vi "Anlagenuebersicht_amium2.vi"() -> ()   [LabVIEW 2020, in "Amium PNS.lvlib"]
uses:
  Amium PNS.lvlib
  PNS Istwerte_Amium.ctl
  Visualisierungs Elemente/String - Ausgabefeld.ctl
  Amium Zustand.ctl
  Seiten/System Einstellungen V2/Aktioen FGV System.ctl
  Aktion FGV Amium Daten.ctl
  Allgemein/allgemeine Sub-VIs.lvlib
  Seiten/System Einstellungen V2/System Einstellungen V2.lvlib
panel:
  in  "Amium Zustände 2":T1 items=["Pause", "Aufheizphase", "Standby", "Messen", "Spülen", "Leakcheck"]
  out "Amium Zustände":T2
  in  "4 - Fach":bool
  in  "10-Fach":bool
  out "IN10":bool caption="TG"
  out "IN10 2":bool caption="Ex"
  out "IN9":bool caption="TG"
  out "IN9 2":bool caption="Ex"
  out "IN8":bool caption="TG"
  out "IN8 2":bool caption="Ex"
  out "IN7":bool caption="TG"
  out "IN7 2":bool caption="Ex"
  out "IN6":bool caption="TG"
  out "IN6 2":bool caption="Ex"
  out "IN3":bool caption="TG"
  out "IN3 2":bool caption="Ex"
  out "IN4":bool caption="TG"
  out "IN4 2":bool caption="Ex"
  out "AA":bool caption="TG"
  out "Purge":bool caption="Ex"
  out "IN5":bool caption="TG"
  out "IN5 2":bool caption="Ex"
  out "IN1":bool caption="TG"
  out "IN1 2":bool caption="Ex"
  out "IN2":bool caption="TG"
  out "IN2 2":bool caption="Ex"
  out "EX":bool caption="TG"
  out "EX2":bool caption="Ex"
  out "PNS Istwerte":T3 {"Istwert 14" format="%.1f"; "Istwert 13" format="%.1f"; "Istwert 12" format="%.1f"; "Istwert 11" format="%.1f"; "Istwert 10" format="%.1f"; "Istwert 9" format="%.1f"; "Istwert 8" format="%.1f"; "Istwert 7" format="%.1f"; "Istwert 6" format="%.1f"; "Istwert 5" format="%.1f"; "Istwert 4" format="%.1f"; "Istwert 3" format="%.1f"; "Istwert 2" format="%.1f"; "Istwert 1" format="%.1f"}
  out "TG2":bool caption="Ex"
  out "TG":bool
  out "Bild":u16(ring)
  # "Pneumatikplan"
  # "Heizkreis 1:"
  # "Heizkreis 2:"
  # "Heizkreis 3:"
  # "Heizkreis 4:"
  # "Heizkreis 5:"
  # "Heizkreis 6:"
  # "Heizkreis 7:"
  # "Heizkreis 8:"
  # "Heizkreis 9:"
  # "Heizkreis 10:"
  # "Ofen / Filter:"
  # "HL Zuleitung:"
  # "Wanddurch-\nführung:"
  # "AddOn"
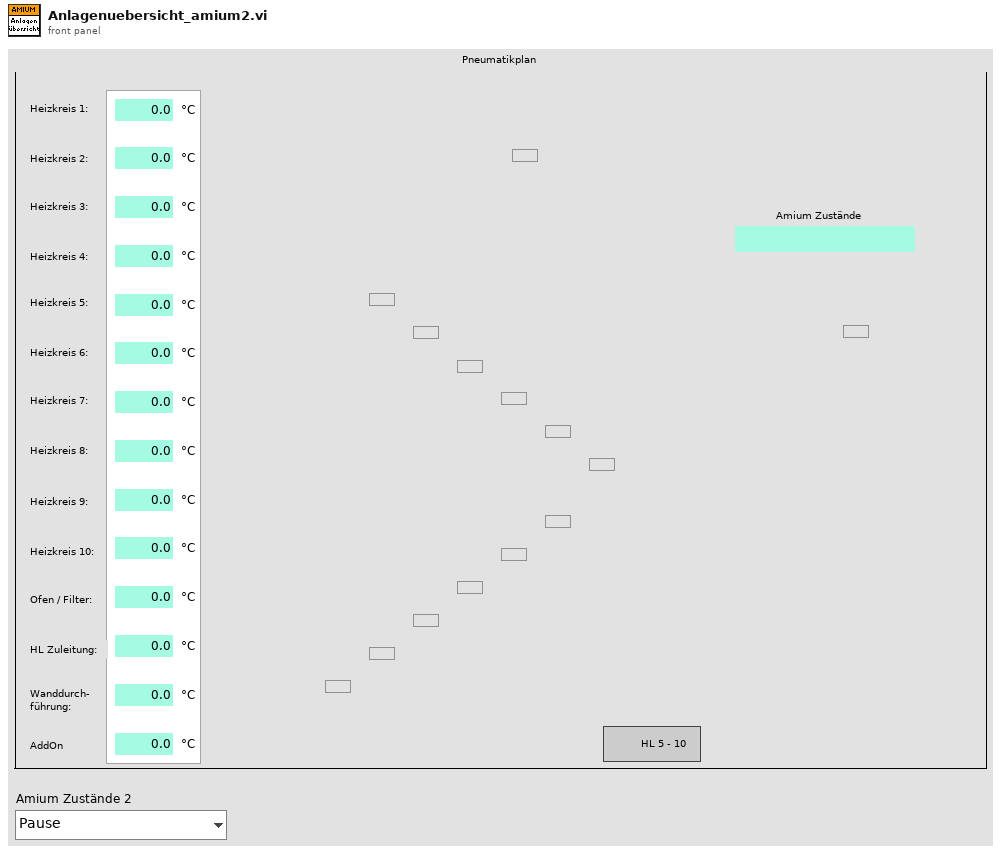
[diagram p1: front panel]
types:
  T1 = typedef "Amium PNS.lvlib/Amium Zustand.ctl" = u16
  T2 = typedef "String - Ausgabefeld.ctl" = string
  T3 = typedef "Amium PNS.lvlib/PNS Istwerte_Amium.ctl" = cluster{"Istwert 1":sgl, "Istwert 2":sgl, "Istwert 3":sgl, "Istwert 4":sgl, "Istwert 5":sgl, "Istwert 6":sgl, "Istwert 7":sgl, "Istwert 8":sgl, "Istwert 9":sgl, "Istwert 10":sgl, "Istwert 11":sgl, "Istwert 12":sgl, "Istwert 13":sgl, "Istwert 14":sgl}
  T4 = typedef "System Einstellungen V2.lvlib/Aktioen FGV System.ctl" = enum16{"lesen", "laden", "speichern", "Optionen schreiben", "Zeitstempel", "Reset BMP", "Reset SQP", "Wartung", "Werkseinstellung"}
  T5 = enum8{"Enabled", "Disabled", "Disabled and Grayed Out"}
  T6 = typedef "System Einstellungen V2.lvlib/Optionen.ctl" = cluster{"Störmeldep.":bool, "Betriebszustände":bool, "AK in ppm":bool, "log Cal-Gas":bool, "log 0-Gas":bool, "Durchflusssensor 0-5V":bool, "PNS?":bool, "Mit N2 spülen":bool, "TRE08":bool, "Amium 10-Fach":bool, "Verticale Scrollbar aktiv":bool, "Loggingtakt":bool, "AK Rezeptwechsel gleich wie MKS":bool, "NG ECO":bool}
  T7 = typedef "Amium PNS.lvlib/Aktion FGV Amium Daten.ctl" = enum16{"lesen", "Komm Daten", "Daten", "Error", "Regler", "Grenzwerte", "laden", "speichern"}
  T8 = typedef "Amium PNS.lvlib/Amium Anlagengrenzwerte PNS.ctl" = cluster{"Filter:":T9, "Ventilplatte:":T9, "Heizleitung 1:":T9, "Heizleitung 2:":T9, "Heizleitung 3:":T9, "Heizleitung 4:":T9, "Heizleitung 5:":T9, "Heizleitung 6:":T9, "Heizleitung 7:":T9, "Heizleitung 8:":T9, "Heizleitung 9:":T9, "Heizleitung 10:":T9, "Heizleitung 11:":T9, "Heizleitung 12:":T9}
  T9 = typedef "Amium PNS.lvlib/Amium Anlagengrenzwerte-Parameter Anzeige.ctl" = cluster{"Sollwert":T10, "Warn-Min":T10, "Warn-Max":T10, "Abschalt-Min":T10, "Abschalt-Max":T10, "Regler":u16}
  T10 = typedef "Zahlen-Eingabefeld.ctl" = sgl
  T11 = typedef "Amium PNS.lvlib/Daten Cluster.ctl" = cluster{"Amium Zustände":T1, "Samplepoint am PNS":i16, "Gerätekennung":string, "aktiver Samplepoint":i16[], "Messgasdruck":sgl}
  T12 = typedef "Amium PNS.lvlib/Temperaturregler Cluster.ctl" = cluster{"Istwert":sgl, "Sollwert":sgl, "Stellgröße":sgl, "Status":sgl, "Error":sgl}
  T13 = cluster{"Istwert":sgl, "Istwert":sgl, "Istwert":sgl, "Istwert":sgl, "Istwert":sgl, "Istwert":sgl, "Istwert":sgl, "Istwert":sgl, "Istwert":sgl, "Istwert":sgl, "Istwert":sgl, "Istwert":sgl, "Istwert":sgl, "Istwert":sgl}
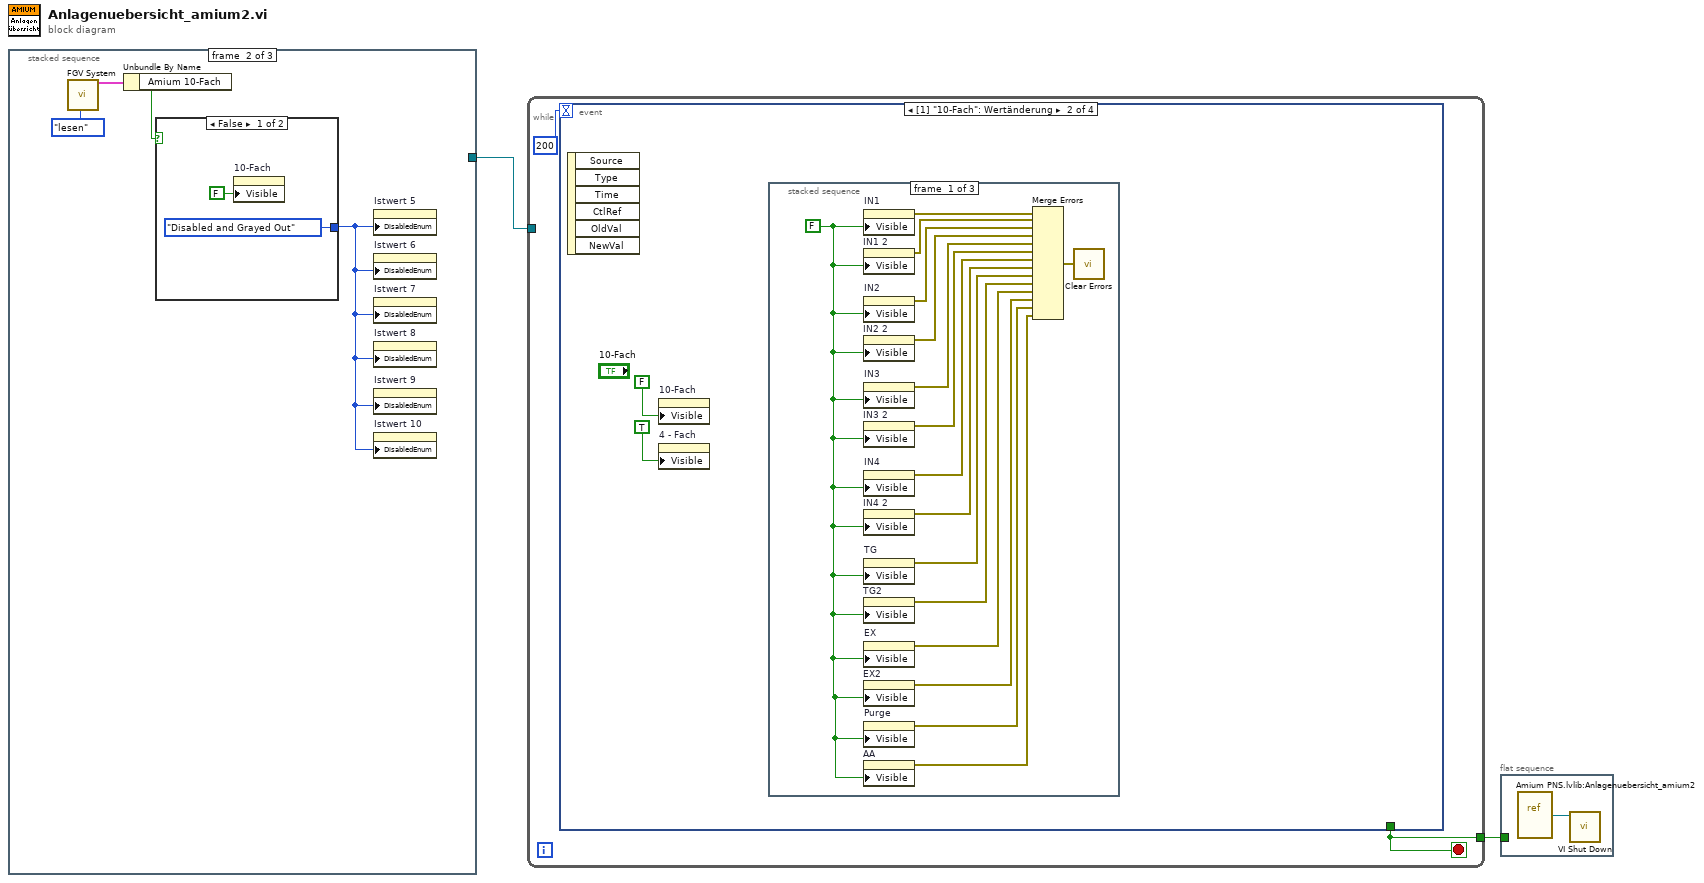
[diagram p0: block diagram]
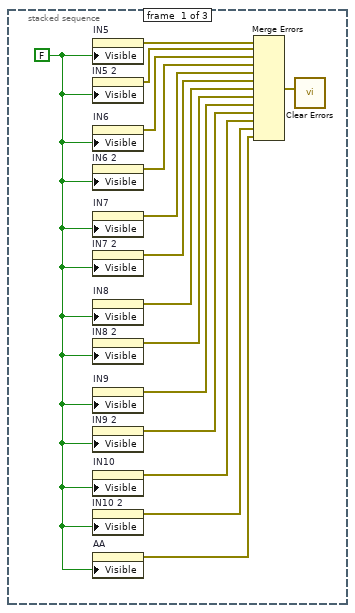
[diagram p2: hidden frame]
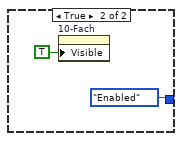
[diagram p3: hidden frame]
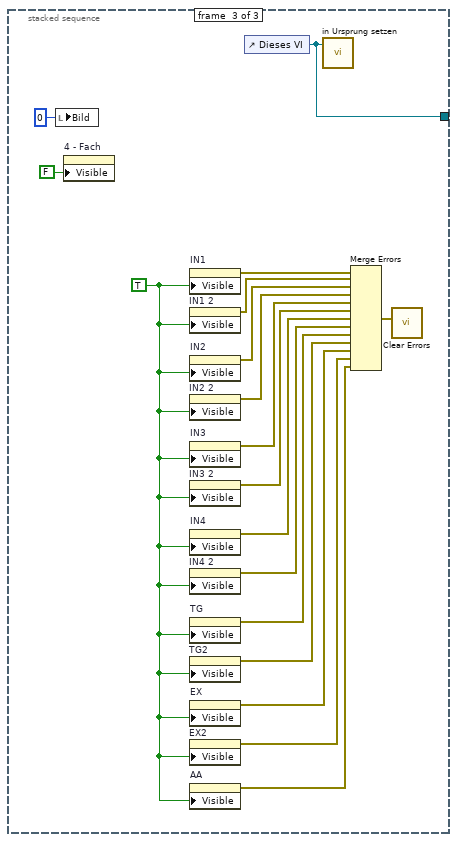
[diagram p4: hidden frame]
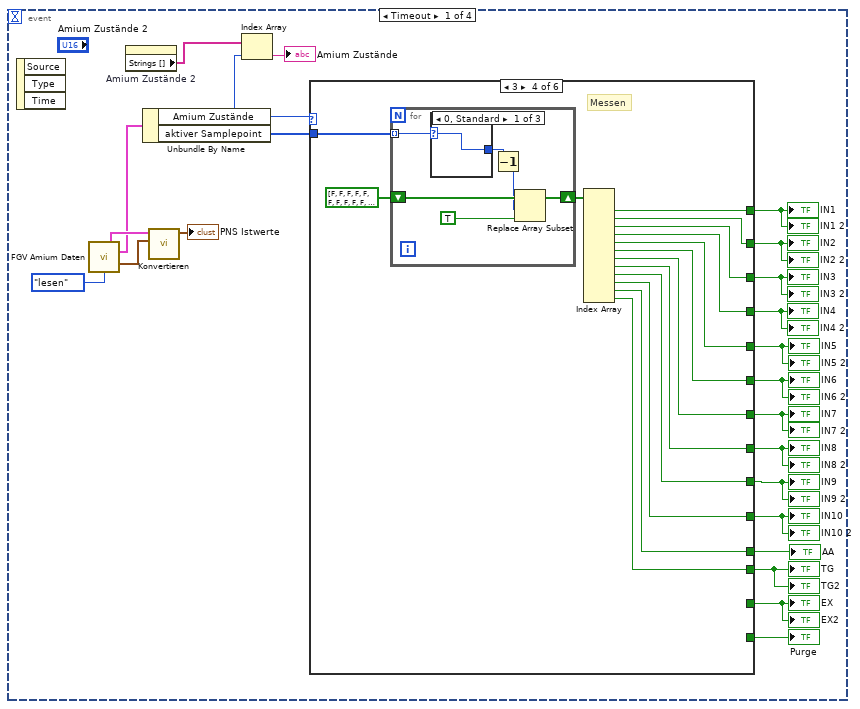
[diagram p5: hidden frame]
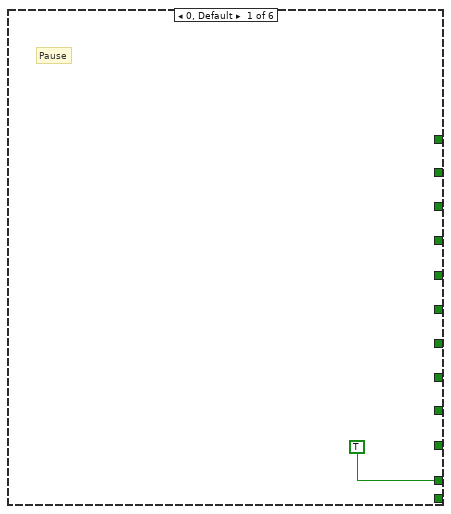
[diagram p6: hidden frame]
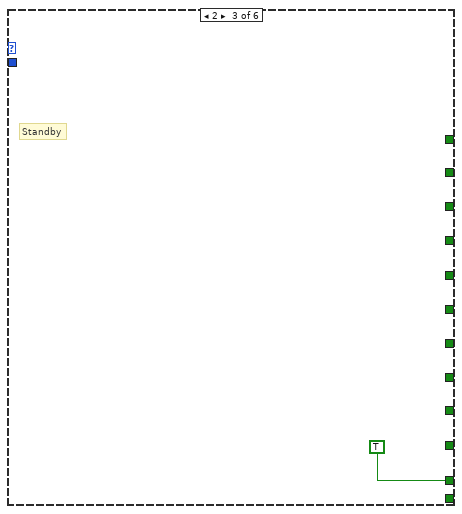
[diagram p8: hidden frame]
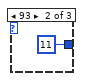
[diagram p9: hidden frame]
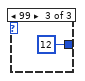
[diagram p10: hidden frame]
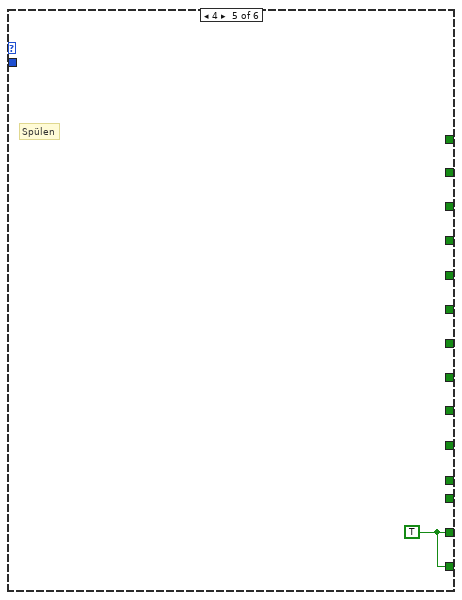
[diagram p11: hidden frame]
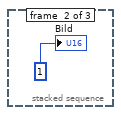
[diagram p13: hidden frame]
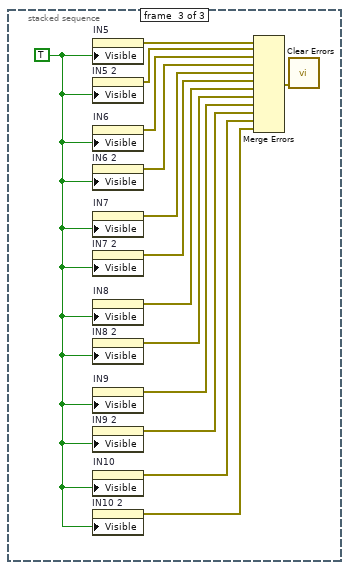
[diagram p14: hidden frame]
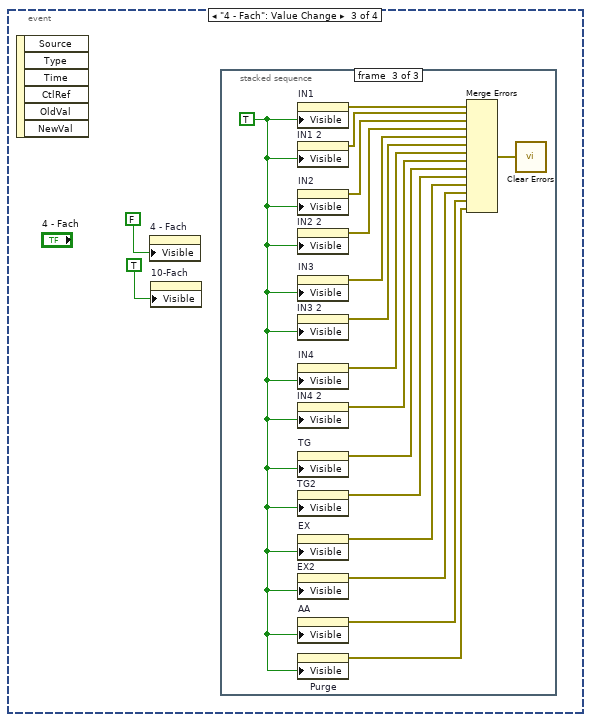
[diagram p15: hidden frame]
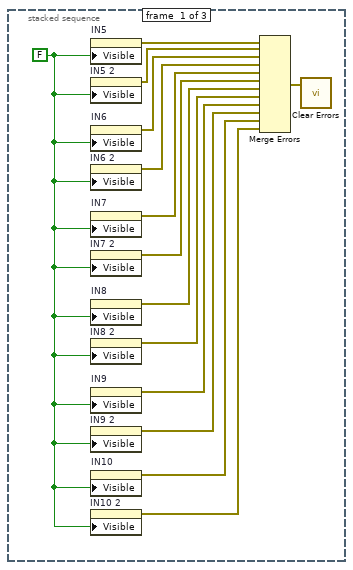
[diagram p16: hidden frame]
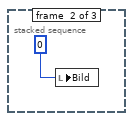
[diagram p17: hidden frame]
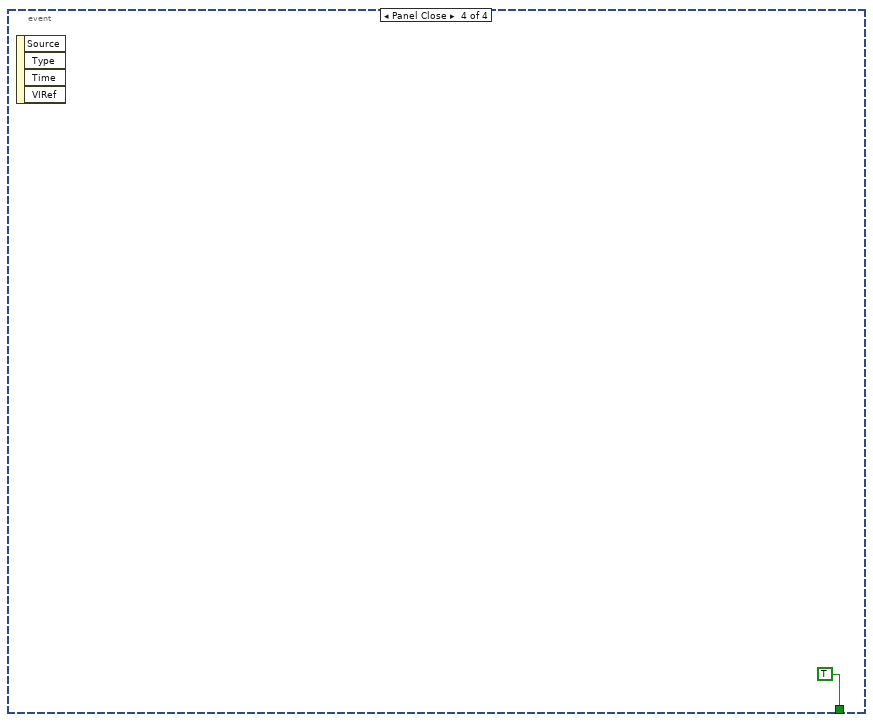
[diagram p18: hidden frame]
diagram:
  n1 = stacked-sequence {
    tunnel: [_ _ w28] -> w2
    frame #0 {
      w4 = FALSE
      n2 = property on="IN5" class="Bool. (strikt)"("Visible"=w4) -> (error out=w5:errorcluster)  [unwired: 2 in, 1 out]
      n3 = property on="IN5 2" class="Bool. (strikt)"("Visible"=w4) -> (error out=w6:errorcluster)  [unwired: 2 in, 1 out]
      n4 = property on="IN6" class="Bool. (strikt)"("Visible"=w4) -> (error out=w7:errorcluster)  [unwired: 2 in, 1 out]
      n5 = property on="IN6 2" class="Bool. (strikt)"("Visible"=w4) -> (error out=w8:errorcluster)  [unwired: 2 in, 1 out]
      n6 = property on="IN7" class="Bool. (strikt)"("Visible"=w4) -> (error out=w9:errorcluster)  [unwired: 2 in, 1 out]
      n7 = property on="IN7 2" class="Bool. (strikt)"("Visible"=w4) -> (error out=w10:errorcluster)  [unwired: 2 in, 1 out]
      n8 = property on="IN8" class="Bool. (strikt)"("Visible"=w4) -> (error out=w11:errorcluster)  [unwired: 2 in, 1 out]
      n9 = property on="IN8 2" class="Bool. (strikt)"("Visible"=w4) -> (error out=w12:errorcluster)  [unwired: 2 in, 1 out]
      n10 = property on="IN9" class="Bool. (strikt)"("Visible"=w4) -> (error out=w13:errorcluster)  [unwired: 2 in, 1 out]
      n11 = property on="IN9 2" class="Bool. (strikt)"("Visible"=w4) -> (error out=w14:errorcluster)  [unwired: 2 in, 1 out]
      n12 = property on="IN10" class="Bool. (strikt)"("Visible"=w4) -> (error out=w15:errorcluster)  [unwired: 2 in, 1 out]
      n13 = property on="IN10 2" class="Bool. (strikt)"("Visible"=w4) -> (error out=w16:errorcluster)  [unwired: 2 in, 1 out]
      n14 = property on="AA" class="Bool. (strikt)"("Visible"=w4) -> (error out=w3:errorcluster)  [unwired: 2 in, 1 out]
      n15 = Merge Errors(w5, w6, w7, w8, w9, w10, w11, w12, w13, w14, w15, w16, w3) -> (w17:errorcluster)
      n16 = call <vilib>:"Clear Errors.vi"("error in (no error)"=w17) -> ()  [unwired: 5 in, 2 out]
    }
    frame #1 {
      n17 = call "FGV System.vi"("Aktionen"=Aktioen_FGV_System."lesen") -> ("Optionen"=w19:T6)  [unwired: 12 in, 6 out]
      n18 = Unbundle By Name(w19) -> ("Amium 10-Fach"=w18:bool)
      n19 = case shown="False" w18 {
        tunnel: [T5."Disabled and Grayed Out" ("Deaktiviert") T5."Enabled" ("Deaktiviert")] -> w21
        frame False {
          n20 = property on="10-Fach" class="Bool."("Visible"=FALSE ("Sichtbar")) -> ()  [unwired: 2 in, 2 out]
        }
        frame True {
          n21 = property on="10-Fach" class="Bool."("Visible"=TRUE ("Sichtbar")) -> ()  [unwired: 2 in, 2 out]
        }
      }
      n22 = property on="Istwert 5" class="DigWert (strikt)"("DisabledEnum"=w21) -> ()  [unwired: 2 in, 2 out]
      n23 = property on="Istwert 6" class="DigWert (strikt)"("DisabledEnum"=w21) -> ()  [unwired: 2 in, 2 out]
      n24 = property on="Istwert 7" class="DigWert (strikt)"("DisabledEnum"=w21) -> ()  [unwired: 2 in, 2 out]
      n25 = property on="Istwert 8" class="DigWert (strikt)"("DisabledEnum"=w21) -> ()  [unwired: 2 in, 2 out]
      n26 = property on="Istwert 9" class="DigWert (strikt)"("DisabledEnum"=w21) -> ()  [unwired: 2 in, 2 out]
      n27 = property on="Istwert 10" class="DigWert (strikt)"("DisabledEnum"=w21) -> ()  [unwired: 2 in, 2 out]
    }
    frame #2 {
      w27 = TRUE
      n28 = local write "Bild"(u16 0 ("Bild")) -> ()
      n29 = property on="4 - Fach" class="Bool."("Visible"=FALSE ("Sichtbar")) -> ()  [unwired: 2 in, 2 out]
      n30 = property on="IN1" class="Bool. (strikt)"("Visible"=w27) -> (error out=w31:errorcluster)  [unwired: 2 in, 1 out]
      n31 = property on="IN1 2" class="Bool. (strikt)"("Visible"=w27) -> (error out=w32:errorcluster)  [unwired: 2 in, 1 out]
      n32 = property on="IN2" class="Bool. (strikt)"("Visible"=w27) -> (error out=w33:errorcluster)  [unwired: 2 in, 1 out]
      n33 = property on="IN2 2" class="Bool. (strikt)"("Visible"=w27) -> (error out=w34:errorcluster)  [unwired: 2 in, 1 out]
      n34 = property on="IN3" class="Bool. (strikt)"("Visible"=w27) -> (error out=w35:errorcluster)  [unwired: 2 in, 1 out]
      n35 = property on="IN3 2" class="Bool. (strikt)"("Visible"=w27) -> (error out=w36:errorcluster)  [unwired: 2 in, 1 out]
      n36 = property on="IN4" class="Bool. (strikt)"("Visible"=w27) -> (error out=w37:errorcluster)  [unwired: 2 in, 1 out]
      n37 = property on="IN4 2" class="Bool. (strikt)"("Visible"=w27) -> (error out=w38:errorcluster)  [unwired: 2 in, 1 out]
      n38 = property on="TG" class="Bool. (strikt)"("Visible"=w27) -> (error out=w39:errorcluster)  [unwired: 2 in, 1 out]
      n39 = property on="TG2" class="Bool. (strikt)"("Visible"=w27) -> (error out=w40:errorcluster)  [unwired: 2 in, 1 out]
      n40 = property on="EX" class="Bool. (strikt)"("Visible"=w27) -> (error out=w41:errorcluster)  [unwired: 2 in, 1 out]
      n41 = property on="EX2" class="Bool. (strikt)"("Visible"=w27) -> (error out=w42:errorcluster)  [unwired: 2 in, 1 out]
      n42 = property on="AA" class="Bool. (strikt)"("Visible"=w27) -> (error out=w26:errorcluster)  [unwired: 2 in, 1 out]
      n43 = control-ref of="Dieses VI"() -> (w28:refnum<vi>)
      n44 = call "in Ursprung setzen.vi"("VI Referenz"=w28) -> ()  [unwired: 10 in, 1 out]
      n45 = Merge Errors(w31, w32, w33, w34, w35, w36, w37, w38, w39, w40, w41, w42, w26) -> (w43:errorcluster)
      n46 = call <vilib>:"Clear Errors.vi"("error in (no error)"=w43) -> ()  [unwired: 5 in, 2 out]
    }
  }
  n47 = while {
    tunnel: w2 -> [_]
    tunnel: [w44] -> w1
    stop <- w44 stop-if-true
    n48 = event shown="[1] \"10-Fach\": Wertänderung" {
      selector: _ -> [_ _ _ _]
      dyn-events: _ -> [_ _ _ _]
      timeout: 200 -> [_ _ _ _]
      tunnel: [_ _ _ TRUE] -> w44
      event Timeout {
        n49 = event-data() -> ()  [unwired: 1 in, 3 out]
        n50 = call "FGV Amium Daten.vi"("Aktion"=Aktion_FGV_Amium_Daten."lesen") -> ("Grenzwerte PNS"=w66:T8, "Amium Daten"=w64:T11, "Regler"=w67:T12[])  [unwired: 9 in, 3 out]
        n51 = property on="Amium Zustände 2" class="Ring (strikt)"() -> ("Strings []"=w46:string[])  [unwired: 2 in, 2 out]
        n52 = Unbundle By Name(w64) -> ("Amium Zustände"=w48:T1, "aktiver Samplepoint"=w49:i16[])
        n53 = call "Konvertieren.vi"("Regler"=w67, "Grenzwerte PNS (Eingang)"=w66) -> ("Cluster"=→"PNS Istwerte":T13)  [unwired: 8 in, 1 out]
        n54 = Index Array(array=w46, index=w48) -> (element=→"Amium Zustände":string)
        n55 = case shown="3" w48 {
          tunnel: w49 -> [_ _ _ w85 _ _]
          tunnel: [_ _ _ w82 _ _] -> w63
          tunnel: [_ _ _ w81 _ _] -> w62
          tunnel: [_ _ _ w80 _ _] -> w59
          tunnel: [_ _ _ w79 _ _] -> w58
          tunnel: [_ _ _ w78 _ _] -> w57
          tunnel: [_ _ _ w77 _ _] -> w56
          tunnel: [_ _ _ w76 _ _] -> w55
          tunnel: [_ _ _ w75 _ _] -> w54
          tunnel: [_ _ _ w74 _ _] -> w53
          tunnel: [_ _ _ w73 _ _] -> w52
          tunnel: [TRUE _ TRUE w72 _ _] -> w61
          tunnel: [_ _ _ w71 _ _] -> w51
          tunnel: [_ _ _ _ w95 _] -> w50
          tunnel: [_ _ _ _ w95 _] -> w60
          frame 0, Default {
            # "Pause"
          }
          frame 1 {
            # "Aufheitzphase"
          }
          frame 2 {
            # "Standby"
          }
          frame 3 {
            # "Messen"
            n56 = for {
              tunnel: w85 -> [w88] mode=indexing
              shift-right: [w90] -> w83
              shift-left: bool[] [FALSE, FALSE, FALSE, FALSE, FALSE, FALSE, FALSE, FALSE, FALSE, FALSE, FALSE, FALSE, FALSE, FALSE, FALSE, FALSE, FALSE, FALSE, FALSE, FALSE, FALSE] ("Array") -> [w89]
              n57 = case shown="0, Standard" w88 {
                selector: w88 -> [w92 _ _]
                tunnel: [w92 i16 11 ("aktiver Samplepoint") i16 12 ("aktiver Samplepoint")] -> w87
                frame 0, Default {
                }
                frame 93 {
                }
                frame 99 {
                }
              }
              n58 = Decrement(x=w87) -> (x-1=w86:i16)
              n59 = Replace Array Subset(array=w89, new element=TRUE, index=w86) -> (w90:bool[])
            }
            n60 = Index Array(array=w83) -> (element #1=w82:bool, element #2=w81:bool, element #3=w80:bool, element #4=w79:bool, element #5=w78:bool, element #6=w77:bool, element #7=w76:bool, element #8=w75:bool, element #9=w74:bool, element #10=w73:bool, element #11=w72:bool, element #12=w71:bool)  [unwired: 12 in]
          }
          frame 4 {
            w95 = TRUE
            # "Spülen"
          }
          frame 5 {
            # "Leakcheck"
          }
        }
        "TG" <- w51
        "TG2" <- w51
        "EX" <- w50
        "EX2" <- w50
        "Purge" <- w60
        "AA" <- w61
        "IN1" <- w63
        "IN1 2" <- w63
        "IN2" <- w62
        "IN2 2" <- w62
        "IN3" <- w59
        "IN3 2" <- w59
        "IN4" <- w58
        "IN4 2" <- w58
        "IN5" <- w57
        "IN5 2" <- w57
        "IN6" <- w56
        "IN6 2" <- w56
        "IN7" <- w55
        "IN7 2" <- w55
        "IN8" <- w54
        "IN8 2" <- w54
        "IN9" <- w53
        "IN9 2" <- w53
        "IN10" <- w52
        "IN10 2" <- w52
      }
      event "10-Fach": Value Change {
        n61 = event-data() -> ()  [unwired: 1 in, 6 out]
        n62 = property on="10-Fach" class="Bool."("Visible"=FALSE ("Sichtbar")) -> ()  [unwired: 2 in, 2 out]
        n63 = property on="4 - Fach" class="Bool."("Visible"=TRUE ("Sichtbar")) -> ()  [unwired: 2 in, 2 out]
        n64 = stacked-sequence {
          frame #0 {
            w100 = FALSE
            n65 = property on="IN1" class="Bool. (strikt)"("Visible"=w100) -> (error out=w113:errorcluster)  [unwired: 2 in, 1 out]
            n66 = property on="IN1 2" class="Bool. (strikt)"("Visible"=w100) -> (error out=w112:errorcluster)  [unwired: 2 in, 1 out]
            n67 = property on="IN2" class="Bool. (strikt)"("Visible"=w100) -> (error out=w111:errorcluster)  [unwired: 2 in, 1 out]
            n68 = property on="IN2 2" class="Bool. (strikt)"("Visible"=w100) -> (error out=w110:errorcluster)  [unwired: 2 in, 1 out]
            n69 = property on="IN3" class="Bool. (strikt)"("Visible"=w100) -> (error out=w109:errorcluster)  [unwired: 2 in, 1 out]
            n70 = property on="IN3 2" class="Bool. (strikt)"("Visible"=w100) -> (error out=w108:errorcluster)  [unwired: 2 in, 1 out]
            n71 = property on="IN4" class="Bool. (strikt)"("Visible"=w100) -> (error out=w107:errorcluster)  [unwired: 2 in, 1 out]
            n72 = property on="IN4 2" class="Bool. (strikt)"("Visible"=w100) -> (error out=w106:errorcluster)  [unwired: 2 in, 1 out]
            n73 = property on="TG" class="Bool. (strikt)"("Visible"=w100) -> (error out=w105:errorcluster)  [unwired: 2 in, 1 out]
            n74 = property on="TG2" class="Bool. (strikt)"("Visible"=w100) -> (error out=w104:errorcluster)  [unwired: 2 in, 1 out]
            n75 = property on="EX" class="Bool. (strikt)"("Visible"=w100) -> (error out=w103:errorcluster)  [unwired: 2 in, 1 out]
            n76 = property on="EX2" class="Bool. (strikt)"("Visible"=w100) -> (error out=w102:errorcluster)  [unwired: 2 in, 1 out]
            n77 = property on="Purge" class="Bool. (strikt)"("Visible"=w100) -> (error out=w99:errorcluster)  [unwired: 2 in, 1 out]
            n78 = property on="AA" class="Bool. (strikt)"("Visible"=w100) -> (error out=w98:errorcluster)  [unwired: 2 in, 1 out]
            n79 = Merge Errors(w113, w112, w111, w110, w109, w108, w107, w106, w105, w104, w103, w102, w99, w98) -> (w101:errorcluster)
            n80 = call <vilib>:"Clear Errors.vi"("error in (no error)"=w101) -> ()  [unwired: 5 in, 2 out]
          }
          frame #1 {
            "Bild" <- u16 1 ("Bild")
          }
          frame #2 {
            w115 = TRUE
            n81 = property on="IN5" class="Bool. (strikt)"("Visible"=w115) -> (error out=w128:errorcluster)  [unwired: 2 in, 1 out]
            n82 = property on="IN5 2" class="Bool. (strikt)"("Visible"=w115) -> (error out=w127:errorcluster)  [unwired: 2 in, 1 out]
            n83 = property on="IN6" class="Bool. (strikt)"("Visible"=w115) -> (error out=w126:errorcluster)  [unwired: 2 in, 1 out]
            n84 = property on="IN6 2" class="Bool. (strikt)"("Visible"=w115) -> (error out=w125:errorcluster)  [unwired: 2 in, 1 out]
            n85 = property on="IN7" class="Bool. (strikt)"("Visible"=w115) -> (error out=w124:errorcluster)  [unwired: 2 in, 1 out]
            n86 = property on="IN7 2" class="Bool. (strikt)"("Visible"=w115) -> (error out=w123:errorcluster)  [unwired: 2 in, 1 out]
            n87 = property on="IN8" class="Bool. (strikt)"("Visible"=w115) -> (error out=w122:errorcluster)  [unwired: 2 in, 1 out]
            n88 = property on="IN8 2" class="Bool. (strikt)"("Visible"=w115) -> (error out=w121:errorcluster)  [unwired: 2 in, 1 out]
            n89 = property on="IN9" class="Bool. (strikt)"("Visible"=w115) -> (error out=w120:errorcluster)  [unwired: 2 in, 1 out]
            n90 = property on="IN9 2" class="Bool. (strikt)"("Visible"=w115) -> (error out=w119:errorcluster)  [unwired: 2 in, 1 out]
            n91 = property on="IN10" class="Bool. (strikt)"("Visible"=w115) -> (error out=w118:errorcluster)  [unwired: 2 in, 1 out]
            n92 = property on="IN10 2" class="Bool. (strikt)"("Visible"=w115) -> (error out=w117:errorcluster)  [unwired: 2 in, 1 out]
            n93 = Merge Errors(w128, w127, w126, w125, w124, w123, w122, w121, w120, w119, w118, w117) -> (w116:errorcluster)
            n94 = call <vilib>:"Clear Errors.vi"("error in (no error)"=w116) -> ()  [unwired: 5 in, 2 out]
          }
        }
      }
      event "4 - Fach": Value Change {
        n95 = event-data() -> ()  [unwired: 1 in, 6 out]
        n96 = property on="4 - Fach" class="Bool."("Visible"=FALSE ("Sichtbar")) -> ()  [unwired: 2 in, 2 out]
        n97 = property on="10-Fach" class="Bool."("Visible"=TRUE ("Sichtbar")) -> ()  [unwired: 2 in, 2 out]
        n98 = stacked-sequence {
          frame #0 {
            w131 = FALSE
            n99 = property on="IN5" class="Bool. (strikt)"("Visible"=w131) -> (error out=w132:errorcluster)  [unwired: 2 in, 1 out]
            n100 = property on="IN5 2" class="Bool. (strikt)"("Visible"=w131) -> (error out=w133:errorcluster)  [unwired: 2 in, 1 out]
            n101 = property on="IN6" class="Bool. (strikt)"("Visible"=w131) -> (error out=w134:errorcluster)  [unwired: 2 in, 1 out]
            n102 = property on="IN6 2" class="Bool. (strikt)"("Visible"=w131) -> (error out=w135:errorcluster)  [unwired: 2 in, 1 out]
            n103 = property on="IN7" class="Bool. (strikt)"("Visible"=w131) -> (error out=w136:errorcluster)  [unwired: 2 in, 1 out]
            n104 = property on="IN7 2" class="Bool. (strikt)"("Visible"=w131) -> (error out=w137:errorcluster)  [unwired: 2 in, 1 out]
            n105 = property on="IN8" class="Bool. (strikt)"("Visible"=w131) -> (error out=w138:errorcluster)  [unwired: 2 in, 1 out]
            n106 = property on="IN8 2" class="Bool. (strikt)"("Visible"=w131) -> (error out=w139:errorcluster)  [unwired: 2 in, 1 out]
            n107 = property on="IN9" class="Bool. (strikt)"("Visible"=w131) -> (error out=w140:errorcluster)  [unwired: 2 in, 1 out]
            n108 = property on="IN9 2" class="Bool. (strikt)"("Visible"=w131) -> (error out=w141:errorcluster)  [unwired: 2 in, 1 out]
            n109 = property on="IN10" class="Bool. (strikt)"("Visible"=w131) -> (error out=w142:errorcluster)  [unwired: 2 in, 1 out]
            n110 = property on="IN10 2" class="Bool. (strikt)"("Visible"=w131) -> (error out=w143:errorcluster)  [unwired: 2 in, 1 out]
            n111 = Merge Errors(w132, w133, w134, w135, w136, w137, w138, w139, w140, w141, w142, w143) -> (w144:errorcluster)
            n112 = call <vilib>:"Clear Errors.vi"("error in (no error)"=w144) -> ()  [unwired: 5 in, 2 out]
          }
          frame #1 {
            n113 = local write "Bild"(u16 0 ("Bild")) -> ()
          }
          frame #2 {
            w148 = TRUE
            n114 = property on="IN1" class="Bool. (strikt)"("Visible"=w148) -> (error out=w149:errorcluster)  [unwired: 2 in, 1 out]
            n115 = property on="IN1 2" class="Bool. (strikt)"("Visible"=w148) -> (error out=w150:errorcluster)  [unwired: 2 in, 1 out]
            n116 = property on="IN2" class="Bool. (strikt)"("Visible"=w148) -> (error out=w151:errorcluster)  [unwired: 2 in, 1 out]
            n117 = property on="IN2 2" class="Bool. (strikt)"("Visible"=w148) -> (error out=w152:errorcluster)  [unwired: 2 in, 1 out]
            n118 = property on="IN3" class="Bool. (strikt)"("Visible"=w148) -> (error out=w153:errorcluster)  [unwired: 2 in, 1 out]
            n119 = property on="IN3 2" class="Bool. (strikt)"("Visible"=w148) -> (error out=w154:errorcluster)  [unwired: 2 in, 1 out]
            n120 = property on="IN4" class="Bool. (strikt)"("Visible"=w148) -> (error out=w155:errorcluster)  [unwired: 2 in, 1 out]
            n121 = property on="IN4 2" class="Bool. (strikt)"("Visible"=w148) -> (error out=w156:errorcluster)  [unwired: 2 in, 1 out]
            n122 = property on="TG" class="Bool. (strikt)"("Visible"=w148) -> (error out=w157:errorcluster)  [unwired: 2 in, 1 out]
            n123 = property on="TG2" class="Bool. (strikt)"("Visible"=w148) -> (error out=w158:errorcluster)  [unwired: 2 in, 1 out]
            n124 = property on="EX" class="Bool. (strikt)"("Visible"=w148) -> (error out=w159:errorcluster)  [unwired: 2 in, 1 out]
            n125 = property on="EX2" class="Bool. (strikt)"("Visible"=w148) -> (error out=w160:errorcluster)  [unwired: 2 in, 1 out]
            n126 = property on="AA" class="Bool. (strikt)"("Visible"=w148) -> (error out=w147:errorcluster)  [unwired: 2 in, 1 out]
            n127 = property on="Purge" class="Bool. (strikt)"("Visible"=w148) -> (error out=w146:errorcluster)  [unwired: 2 in, 1 out]
            n128 = Merge Errors(w149, w150, w151, w152, w153, w154, w155, w156, w157, w158, w159, w160, w147, w146) -> (w161:errorcluster)
            n129 = call <vilib>:"Clear Errors.vi"("error in (no error)"=w161) -> ()  [unwired: 5 in, 2 out]
          }
        }
      }
      event Panel Close {
        n130 = event-data() -> ()  [unwired: 1 in, 4 out]
      }
    }
  }
  n131 = flat-sequence {
    tunnel: w1 -> [_]
    frame #0 {
      n132 = vi-ref "Amium PNS.lvlib:Anlagenuebersicht_amium2.vi"() -> (w163:refnum<vi>)
      n133 = call "VI Shut Down.vi"("VI Referenz"=w163) -> ()  [unwired: 11 in]
    }
  }
